vi "Read Transfer by ID.vi"(8 "error in (no error)":errorcluster, 10 "Transfer ID":string, 11 "Configuration Session in":refnum<class "Configuration Session.lvclass">) -> (0 "error out":errorcluster, 1 "value":T1, 3 "Configuration Session out":refnum<class "Configuration Session.lvclass">, 4 "found?":bool)   [LabVIEW 2017, in "DSF Core.lvlib" / "Configuration Session.lvclass"]
doc: "Reads a value associated with a key in a specified section from the configuration data identified by <B>dsf refnum</B>. If the key does not exist, the VI returns the default value. This VI supports multibyte characters in strings. Wire data to the <B>default value</B> input to determine the polymorphic instance to use or manually select the instance."
uses:
  Configuration Session.lvclass
  Typedefs/DSF Transfer Info.ctl
  Typedefs/DSF Byte Order.ctl
  Configuration Session.lvclass/Configuration Session.ctl
  DSF Core.lvlib
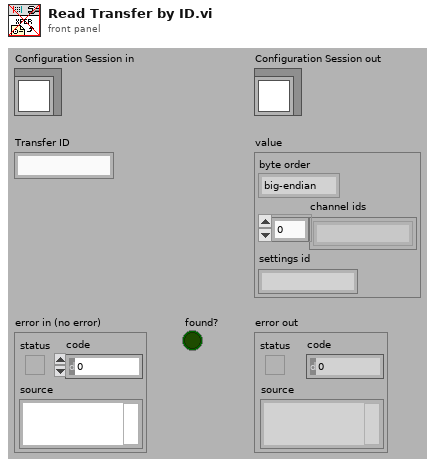
[diagram p1: front panel]
types:
  T1 = typedef "DSF Core.lvlib/DSF Transfer Info.ctl" = cluster{"byte order":T2, "channel ids":string[], "settings id":string}
  T2 = typedef "DSF Core.lvlib/DSF Byte Order.ctl" = enum8{"big-endian", "little-endian"}
  T3 = typedef "DSF Core.lvlib/Configuration Session.lvclass/DSF Config Data Ref.ctl" = refnum<data-value>
  T4 = typedef "DSF Core.lvlib/Configuration Session.lvclass/DSF Config Data.ctl" = cluster{"dsf configuration":T5, "path":path, "dirty":bool}
  T5 = typedef "DSF Core.lvlib/Configuration Session.lvclass/Internal DSF Configuration.ctl" = cluster{"dsfversion":T6, "version":T6, "plugins":T7[], "groups":T12[], "transfers":T14[], "channels":T16[], "settings":T18[], "framework configuration":T20}
  T6 = typedef "DSF Core.lvlib/DSF Version Info.ctl" = cluster{"major":u32, "minor":u32, "fix":u32, "build":string}
  T7 = typedef "DSF Core.lvlib/Configuration Session.lvclass/Internal DSF Plugin with ID.ctl" = cluster{"id":string, "values":T8}
  T8 = typedef "DSF Core.lvlib/Configuration Session.lvclass/Internal DSF Plugin Info.ctl" = cluster{"components":string[], "timing":T9, "group ids":string[], "settings id":string, "threads":T10[]}
  T9 = typedef "DSF Core.lvlib/DSF Timing Info.ctl" = cluster{"priority":u64, "decimation":u64, "offset":u64}
  T10 = typedef "DSF Core.lvlib/DSF Engine Plugin Thread Configuration.ctl" = cluster{"buffer converter settings":T11, "transceiver settings":T11, "custom settings":T11, "processor":i32, "priority offset":i16}
  T11 = typedef "DSF Core.lvlib/DSF Settings Info.ctl" = cluster{"key":string, "value":string}[]
  T12 = typedef "DSF Core.lvlib/Configuration Session.lvclass/Internal DSF Group with ID.ctl" = cluster{"id":string, "values":T13}
  T13 = typedef "DSF Core.lvlib/Configuration Session.lvclass/Internal DSF Group Info.ctl" = cluster{"direction":i32, "timing":T9, "transfer ids":string[], "settings id":string, "thread":i32, "timeout behavior":u8}
  T14 = typedef "DSF Core.lvlib/Configuration Session.lvclass/Internal DSF Transfer with ID.ctl" = cluster{"id":string, "values":T15}
  T15 = typedef "DSF Core.lvlib/Configuration Session.lvclass/Internal DSF Transfer Info.ctl" = cluster{"byte order":i32, "channel ids":string[], "settings id":string}
  T16 = typedef "DSF Core.lvlib/Configuration Session.lvclass/Internal DSF Channel with ID.ctl" = cluster{"id":string, "values":T17}
  T17 = typedef "DSF Core.lvlib/Configuration Session.lvclass/Internal DSF Channel Info.ctl" = cluster{"string buffer offset":u64, "string data type":i32, "engine data type":i32, "settings id":string, "units":string}
  T18 = typedef "DSF Core.lvlib/Configuration Session.lvclass/Internal DSF Settings with ID.ctl" = cluster{"id":string, "values":T19}
  T19 = typedef "DSF Core.lvlib/Configuration Session.lvclass/Internal DSF Settings Info.ctl" = cluster{"key":string, "value":string}[]
  T20 = typedef "DSF Core.lvlib/DSF Engine Framework Configuration.ctl" = cluster{"Plugins":T21[]}
  T21 = typedef "DSF Core.lvlib/DSF Engine Plugin Configuration.ctl" = cluster{"name":string, "components":string[], "cycle timing":T9, "threads":T10[], "Transfer Groups":T22[], "settings":T11}
  T22 = typedef "DSF Core.lvlib/DSF Engine Transfer Group Configuration.ctl" = cluster{"name":string, "direction":T23, "cycle timing":T9, "thread index":i32, "settings":T11, "Transfers":T24[], "timeout behavior":T27}
  T23 = typedef "DSF Core.lvlib/DSF Direction.ctl" = enum8{"Tx", "Rx"}
  T24 = typedef "DSF Core.lvlib/DSF Engine Transfer Configuration.ctl" = cluster{"name":string, "byte order":T2, "settings":T11, "channels":T25[]}
  T25 = typedef "DSF Core.lvlib/DSF Engine Channel Configuration.ctl" = cluster{"string offset":u64, "string data type":T26, "engine data type":T26, "name":string, "settings":T11, "units":string}
  T26 = typedef "DSF Core.lvlib/DSF Data Type.ctl" = enum8{"Bool", "SGL", "DBL", "I8", "I16", "I32", "I64", "U8", "U16", "U32", "U64"}
  T27 = typedef "DSF Core.lvlib/DSF Timeout Behavior.ctl" = enum8{"Increment Late Count", "Throw Error"}
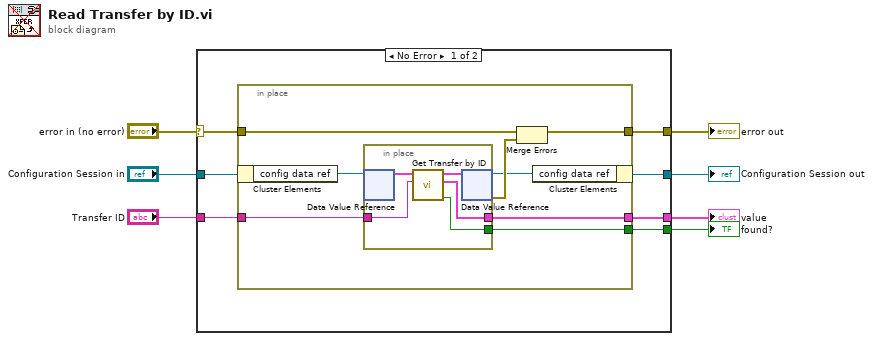
[diagram p0: block diagram]
diagram:
  n1 = case shown="No Error" "error in (no error)" {
    selector: "error in (no error)" -> [w8 w28]
    tunnel: [w14 w28] -> w7
    tunnel: "Transfer ID" -> [w13 _]
    tunnel: [w12 _] -> w5
    tunnel: [w11 _] -> w4
    tunnel: "Configuration Session in" -> [w10 w29]
    tunnel: [w9 w29] -> w2
    frame No Error {
      n2 = in-place {
        in-place-border: w8 -> [w22]
        in-place-border: [w21] -> w14
        in-place-border: w13 -> [w20]
        in-place-border: [w19] -> w12
        in-place-border: [w17] -> w11
        n3 = in-place-cluster #1(w10) -> ("config data ref"=w16:T3)
        n4 = in-place {
          in-place-border: w20 -> [w27]
          in-place-border: [w26] -> w17
          in-place-border: [w25] -> w19
          n5 = in-place-dvr #2(w16) -> (w24:T4)  [unwired: 1 out]
          n6 = call "Get Transfer by ID.vi"("id"=w27, "DSF Configuration in"=w24) -> ("exists?"=w25:bool, "info"=w26:T1, "DSF Configuration out"=w23:T4)  [unwired: 6 in, 1 out]
          n7 = in-place-dvr #2(w23) -> (w15:T3, w18:errorcluster)
        }
        n8 = Merge Errors(w22, w18) -> (w21:errorcluster)
        n9 = in-place-cluster #1("config data ref"=w15) -> (w9:refnum<class "Configuration Session.lvclass">)
      }
    }
    frame Error {
    }
  }
  "error out" <- w7
  "found?" <- w5
  "value" <- w4
  "Configuration Session out" <- w2
